vi "Temperature Status.vi"(8 "error in (no error)":errorcluster, 11 "Cooler in":refnum<class "Cooler.lvclass">) -> (0 "error out":errorcluster, 3 "Cooler out":refnum<class "Cooler.lvclass">)   [LabVIEW 2018, in "Cooler.lvclass"]
doc: "Este VI realiza a leitura da temperatura real do CCD e do status da temperatura, escrevendo estes valores na classe."
uses:
  Cooler.lvclass
  Cooler.lvclass/Cooler.ctl
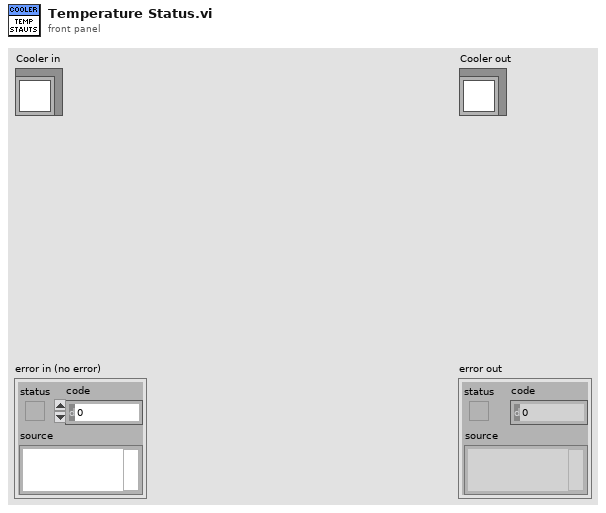
[diagram p1: front panel]
types:
  T1 = typedef "Error Code Enum typedef.ctl" = enum32{"N/A (0)", "DRV_ERROR_CODES", "DRV_SUCCESS", "DRV_VXDNOTINSTALLED", "DRV_ERROR_SCAN", "DRV_ERROR_CHECK_SUM", "DRV_ERROR_FILELOAD", "DRV_UNKNOWN_FUNC", "DRV_ERROR_VXD_INIT", "DRV_ERROR_ADDRESS", "DRV_ERROR_PAGELOCK", "DRV_ERROR_PAGEUNLOCK", "DRV_ERROR_BOARDTEST", "DRV_ERROR_ACK", "DRV_ERROR_UP_FIFO", "DRV_ERROR_PATTERN", "N/A (16)", "DRV_ACQUISITION_ERRORS", "DRV_ACQ_BUFFER", "DRV_ACQ_DOWNFIFO_FULL", "DRV_PROC_UNKONWN_INSTRUCTION", "DRV_ILLEGAL_OP_CODE", "DRV_KINETIC_TIME_NOT_MET", "DRV_ACCUM_TIME_NOT_MET", "DRV_NO_NEW_DATA", "N/A (25)", "DRV_SPOOLERROR", "N/A (27)", "N/A (28)", "N/A (29)", "N/A (30)", "N/A (31)", "N/A (32)", "DRV_TEMPERATURE_CODES", "DRV_TEMPERATURE_OFF", "DRV_TEMPERATURE_NOT_STABILIZED", "DRV_TEMPERATURE_STABILIZED", "DRV_TEMPERATURE_NOT_REACHED", "DRV_TEMPERATURE_OUT_RANGE", "DRV_TEMPERATURE_NOT_SUPPORTED", "DRV_TEMPERATURE_DRIFT", "N/A (41)", "N/A (42)", "N/A (43)", "N/A (44)", "N/A (45)", "N/A (46)", "N/A (47)", "N/A (48)", "DRV_GENERAL_ERRORS", "DRV_INVALID_AUX", "DRV_COF_NOTLOADED", "DRV_FPGAPROG", "DRV_FLEXERROR", "DRV_GPIBERROR", "N/A (55)", "N/A (56)", "N/A (57)", "N/A (58)", "N/A (59)", "N/A (60)", "N/A (61)", "N/A (62)", "N/A (63)", "DRV_DATATYPE", "DRV_DRIVER_ERRORS", "DRV_P1INVALID", "DRV_P2INVALID", "DRV_P3INVALID", "DRV_P4INVALID", "DRV_INIERROR", "DRV_COFERROR", "DRV_ACQUIRING", "DRV_IDLE", "DRV_TEMPCYCLE", "DRV_NOT_INITIALIZED", "DRV_P5INVALID", "DRV_P6INVALID", "DRV_INVALID_MODE", "DRV_INVALID_FILTER", "DRV_I2CERRORS", "DRV_I2CDEVNOTFOUND", "DRV_I2CTIMEOUT", "DRV_P7INVALID", "N/A (84)", "N/A (85)", "N/A (86)", "N/A (87)", "N/A (88)", "N/A (89)", "DRV_IOCERROR", "DRV_VRMVERSIONERROR"}
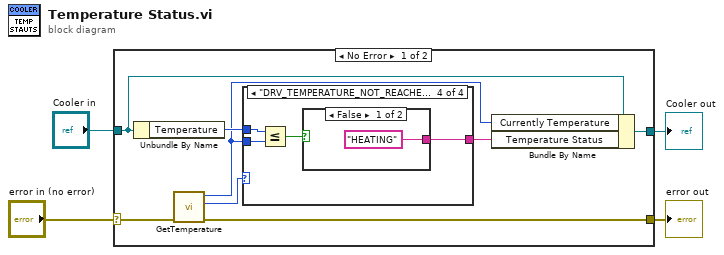
[diagram p0: block diagram]
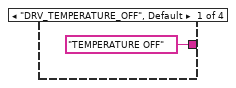
[diagram p2: hidden frame]
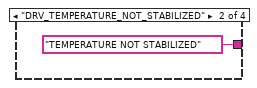
[diagram p3: hidden frame]
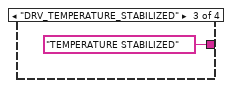
[diagram p4: hidden frame]
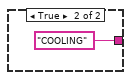
[diagram p5: hidden frame]
diagram:
  n1 = case shown="No Error" "error in (no error)" {
    selector: "error in (no error)" -> [w6 w23]
    tunnel: [w7 w23] -> w1
    tunnel: [w10 w22] -> w2
    tunnel: "Cooler in" -> [w5 w22]
    frame No Error {
      n2 = Unbundle By Name(w5) -> ("Temperature"=w11:i8)
      n3 = call <userlib>:"GetTemperature.vi"("error in (no error)"=w6) -> ("error out"=w7:errorcluster, "status"=w12:T1, "temperature"=w8:i32)  [unwired: 3 in, 1 out]
      n4 = case shown="\"DRV_TEMPERATURE_NOT_REACHED\"" w12 {
        tunnel: ["TEMPERATURE OFF" "TEMPERATURE NOT STABILIZED" "TEMPERATURE STABILIZED" w16] -> w9
        tunnel: w11 -> [_ _ _ w19]
        tunnel: w8 -> [_ _ _ w18]
        frame "DRV_TEMPERATURE_OFF", Default {
        }
        frame "DRV_TEMPERATURE_NOT_STABILIZED" {
        }
        frame "DRV_TEMPERATURE_STABILIZED" {
        }
        frame "DRV_TEMPERATURE_NOT_REACHED" {
          n5 = Less Or Equal?(x=w19, y=w18) -> (x <= y?=w17:bool)
          n6 = case shown="False" w17 {
            tunnel: ["HEATING" "COOLING"] -> w16
            frame False {
            }
            frame True {
            }
          }
        }
      }
      n7 = Bundle By Name(cluster=w5, "Currently Temperature"=w8, "Temperature Status"=w9) -> (w10:refnum<class "Cooler.lvclass">)
    }
    frame Error {
    }
  }
  "error out" <- w1
  "Cooler out" <- w2
